vi "Setting.vi"() -> ()   [LabVIEW 2020]
uses:
  Libraries/S7/S7.lvlib
  <userlib>/_MGI/1D Array/MGI Average/MGI Average (DBL[]).vi
panel:
  in  "输出轴大量程标定":bool
  in  "停止":bool
  in  "输出轴小量程标定":bool
  in  "输入轴标定":bool
  out "标定曲线":cluster{dbl[], dbl[]}[](graph)
  # "配置标定"
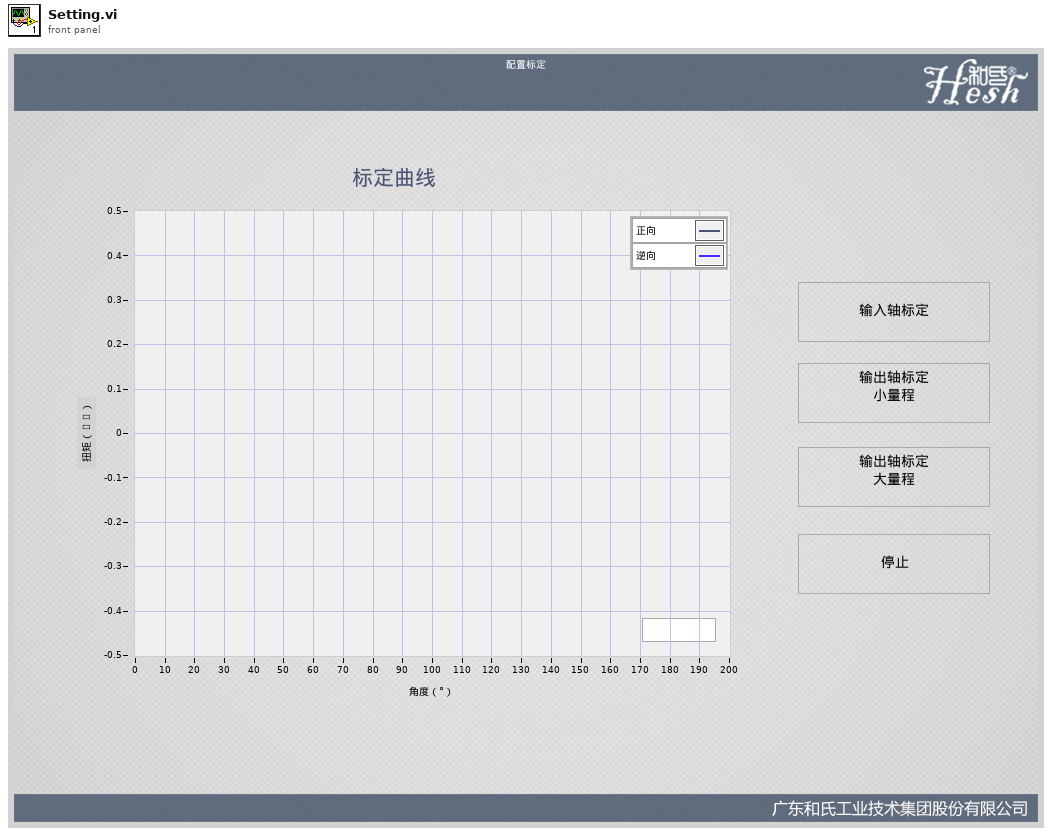
[diagram p1: front panel]
types:
  T1 = cluster{"输入旋转位移":sgl, "输入移载位移":sgl, "工装移载位移":sgl, "输入编码位移":sgl, "输入扭矩":sgl, "输出扭矩(小)":sgl, "输出扭矩(大)":sgl, "吸收电流":sgl}
  T2 = cluster{"输入轴扭矩":dbl, "输出轴扭矩小量程":dbl, "输出轴扭矩大量程":dbl}
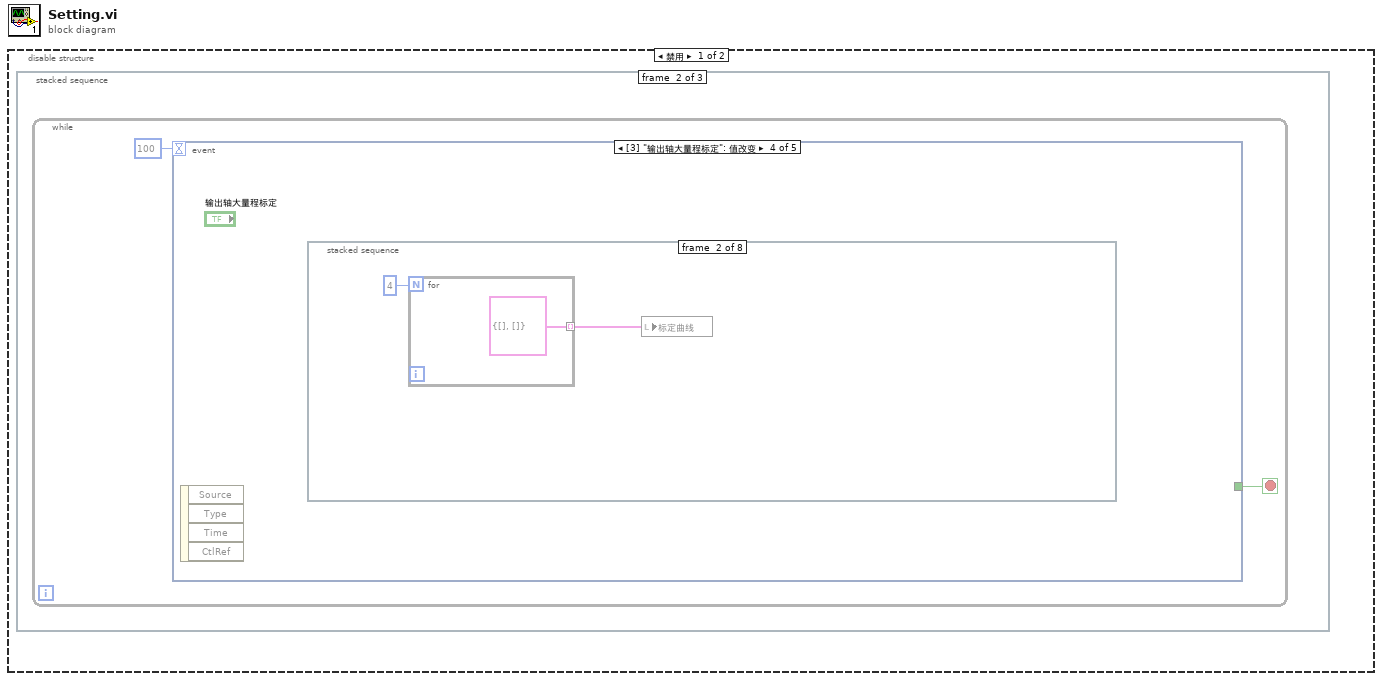
[diagram p0: block diagram]
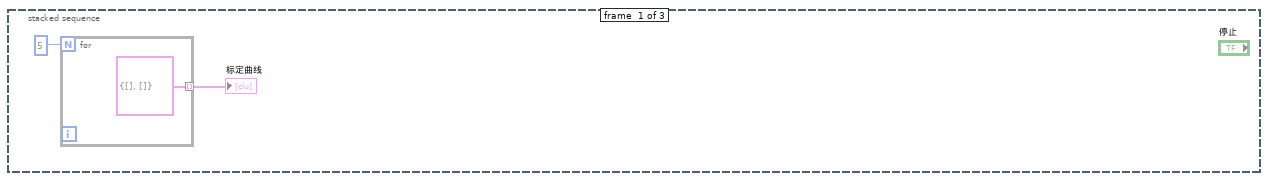
[diagram p2: hidden frame]
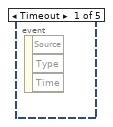
[diagram p3: hidden frame]
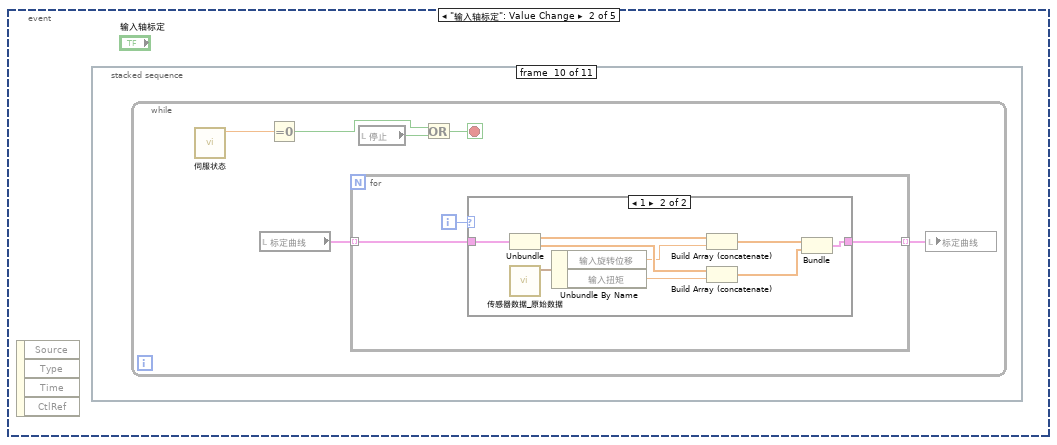
[diagram p4: hidden frame]
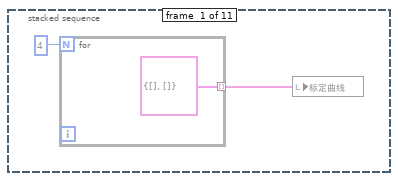
[diagram p5: hidden frame]
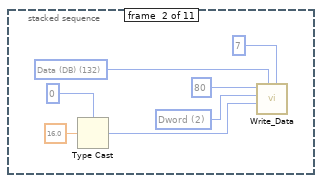
[diagram p6: hidden frame]
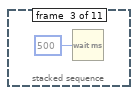
[diagram p7: hidden frame]
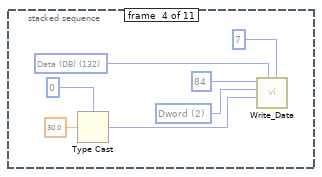
[diagram p8: hidden frame]
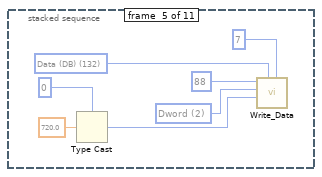
[diagram p9: hidden frame]
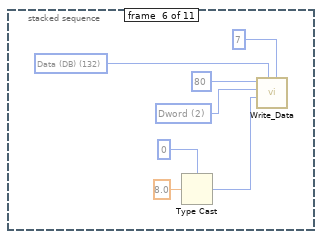
[diagram p10: hidden frame]
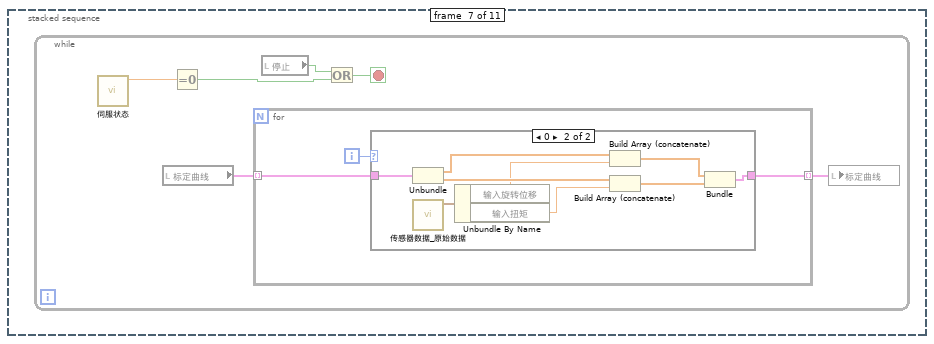
[diagram p11: hidden frame]
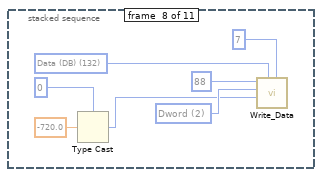
[diagram p13: hidden frame]
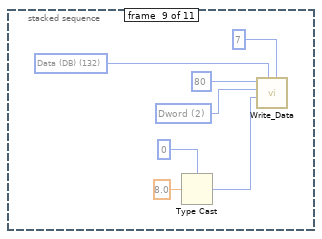
[diagram p14: hidden frame]
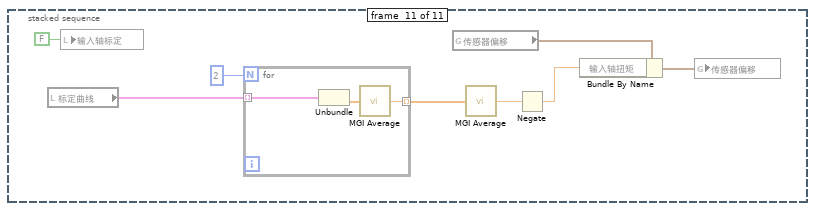
[diagram p16: hidden frame]
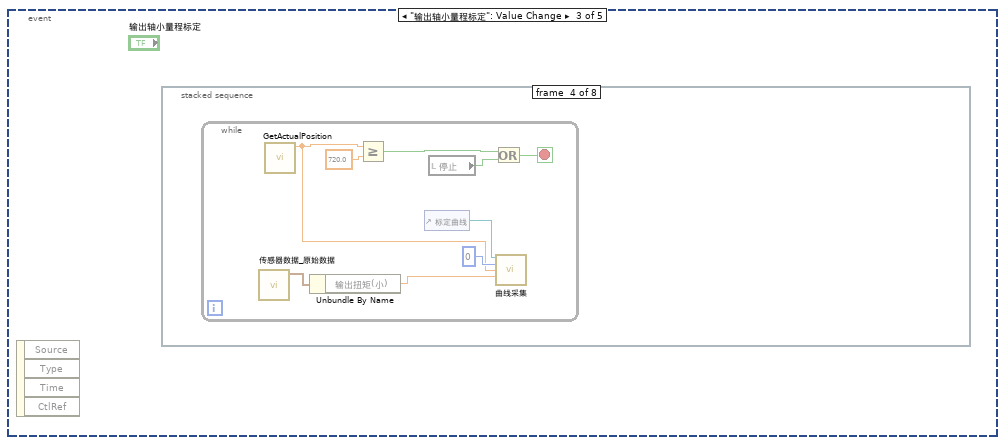
[diagram p17: hidden frame]
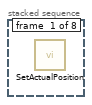
[diagram p18: hidden frame]
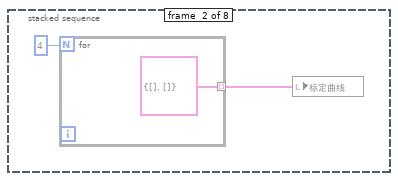
[diagram p19: hidden frame]
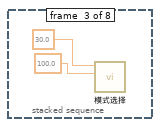
[diagram p20: hidden frame]
diagram:
  n1 = disable-structure shown="禁用" {
    frame Disabled {
      n2 = stacked-sequence {
        frame #0 {
          n3 = for {
            N: 5 -> [_]
            tunnel: [cluster{dbl[], dbl[]} {[], []}] -> w1 mode=indexing
          }
          "标定曲线" <- w1
        }
        frame #1 {
          n4 = while {
            stop <- w5 stop-if-true
            n5 = event shown="[3] \"输出轴大量程标定\": 值改变" {
              selector: _ -> [_ _ _ _ _]
              dyn-events: _ -> [_ _ _ _ _]
              timeout: 100 -> [_ _ _ _ _]
              tunnel: [_ _ _ _ TRUE] -> w5
              event Timeout {
                n6 = event-data() -> ()  [unwired: 1 in, 3 out]
              }
              event "输入轴标定": Value Change {
                n7 = event-data() -> ()  [unwired: 1 in, 4 out]
                n8 = stacked-sequence {
                  frame #0 {
                    n9 = for {
                      N: 4 -> [_]
                      tunnel: [cluster{dbl[], dbl[]} {[], []}] -> w7 mode=indexing
                    }
                    n10 = local write "标定曲线"(w7) -> ()
                  }
                  frame #1 {
                    w13 = u16 2 items=["byte", "word", "Dword"] ("数据类型")
                    w15 = u8 132 items=["I/O (P)"=128, "Input (I)"=129, "Output (Q)"=130, "Bit Memory (M)"=131, "Data (DB)"=132, "Instance Data (DI)"=133, "Local Data (L)"=134, "Predecessor Local Data (VL)"=135] ("寄存器类型")
                    n11 = Type Cast(type=u32 0, x=sgl 16.0 ("输入轴旋转绝对位置")) -> (*(type *) &x=w11:u32)
                    n12 = call "Write_Data.vi"("DB #"=u16 7, "寄存器类型"=w15, "写入数据"=w11, "数据类型"=w13, "写入地址"=u32 80) -> ()  [unwired: 4 in, 3 out]
                  }
                  frame #2 {
                    n13 = Wait (ms)(milliseconds to wait=u32 500 ("等待时间（毫秒）")) -> ()  [unwired: 1 out]
                  }
                  frame #3 {
                    w21 = u16 2 items=["byte", "word", "Dword"] ("数据类型")
                    w23 = u8 132 items=["I/O (P)"=128, "Input (I)"=129, "Output (Q)"=130, "Bit Memory (M)"=131, "Data (DB)"=132, "Instance Data (DI)"=133, "Local Data (L)"=134, "Predecessor Local Data (VL)"=135] ("寄存器类型")
                    n14 = Type Cast(type=u32 0, x=sgl 30.0 ("输入轴旋转绝对位置")) -> (*(type *) &x=w19:u32)
                    n15 = call "Write_Data.vi"("DB #"=u16 7, "寄存器类型"=w23, "写入数据"=w19, "数据类型"=w21, "写入地址"=u32 84) -> ()  [unwired: 4 in, 3 out]
                  }
                  frame #4 {
                    w27 = u16 2 items=["byte", "word", "Dword"] ("数据类型")
                    w28 = u8 132 items=["I/O (P)"=128, "Input (I)"=129, "Output (Q)"=130, "Bit Memory (M)"=131, "Data (DB)"=132, "Instance Data (DI)"=133, "Local Data (L)"=134, "Predecessor Local Data (VL)"=135] ("寄存器类型")
                    n16 = Type Cast(type=u32 0, x=sgl 720.0 ("输入轴旋转绝对位置")) -> (*(type *) &x=w30:u32)
                    n17 = call "Write_Data.vi"("DB #"=u16 7, "寄存器类型"=w28, "写入数据"=w30, "数据类型"=w27, "写入地址"=u32 88) -> ()  [unwired: 4 in, 3 out]
                  }
                  frame #5 {
                    w34 = u16 2 items=["byte", "word", "Dword"] ("数据类型")
                    w35 = u8 132 items=["I/O (P)"=128, "Input (I)"=129, "Output (Q)"=130, "Bit Memory (M)"=131, "Data (DB)"=132, "Instance Data (DI)"=133, "Local Data (L)"=134, "Predecessor Local Data (VL)"=135] ("寄存器类型")
                    n18 = Type Cast(type=u32 0, x=sgl 8.0 ("输入轴旋转绝对位置")) -> (*(type *) &x=w37:u32)
                    n19 = call "Write_Data.vi"("DB #"=u16 7, "寄存器类型"=w35, "写入数据"=w37, "数据类型"=w34, "写入地址"=u32 80) -> ()  [unwired: 4 in, 3 out]
                  }
                  frame #6 {
                    n20 = while {
                      stop <- w42 stop-if-true
                      n21 = call "伺服状态.vi"() -> ("Status"=w39:sgl)  [unwired: 11 in]
                      n22 = local read "标定曲线"() -> (w41:cluster{dbl[], dbl[]}[])
                      n23 = Equal To 0?(x=w39) -> (x = 0?=w38:bool)
                      n24 = for {
                        tunnel: [w44] -> w40 mode=indexing
                        tunnel: w41 -> [w46] mode=indexing
                        i -> [w45]
                        n25 = case shown="0" w45 {
                          tunnel: [w47 w51] -> w44
                          tunnel: w46 -> [w47 w52]
                          frame Default {
                          }
                          frame 0 {
                            n26 = Unbundle(w52) -> (w56:dbl[], w55:dbl[])
                            n27 = call "传感器数据_原始数据.vi"() -> ("传感器读数"=w50:T1)  [unwired: 11 in]
                            n28 = Unbundle By Name(w50) -> ("输入旋转位移"=w49:sgl, "输入扭矩"=w48:sgl)
                            n29 = Build Array (concatenate)(w56, w49) -> (w54:dbl[])
                            n30 = Build Array (concatenate)(w55, w48) -> (w53:dbl[])
                            n31 = Bundle(w54, w53) -> (w51:cluster{dbl[], dbl[]})  [unwired: 1 in]
                          }
                        }
                      }
                      n32 = local read "停止"() -> (w43:bool)
                      n33 = Or(x=w43, y=w38) -> (x .or. y?=w42:bool)
                      n34 = local write "标定曲线"(w40) -> ()
                    }
                  }
                  frame #7 {
                    w61 = u16 2 items=["byte", "word", "Dword"] ("数据类型")
                    w63 = u8 132 items=["I/O (P)"=128, "Input (I)"=129, "Output (Q)"=130, "Bit Memory (M)"=131, "Data (DB)"=132, "Instance Data (DI)"=133, "Local Data (L)"=134, "Predecessor Local Data (VL)"=135] ("寄存器类型")
                    n35 = Type Cast(type=u32 0, x=sgl -720.0 ("输入轴旋转绝对位置")) -> (*(type *) &x=w59:u32)
                    n36 = call "Write_Data.vi"("DB #"=u16 7, "寄存器类型"=w63, "写入数据"=w59, "数据类型"=w61, "写入地址"=u32 88) -> ()  [unwired: 4 in, 3 out]
                  }
                  frame #8 {
                    w68 = u16 2 items=["byte", "word", "Dword"] ("数据类型")
                    w70 = u8 132 items=["I/O (P)"=128, "Input (I)"=129, "Output (Q)"=130, "Bit Memory (M)"=131, "Data (DB)"=132, "Instance Data (DI)"=133, "Local Data (L)"=134, "Predecessor Local Data (VL)"=135] ("寄存器类型")
                    n37 = Type Cast(type=u32 0, x=sgl 8.0 ("输入轴旋转绝对位置")) -> (*(type *) &x=w66:u32)
                    n38 = call "Write_Data.vi"("DB #"=u16 7, "寄存器类型"=w70, "写入数据"=w66, "数据类型"=w68, "写入地址"=u32 80) -> ()  [unwired: 4 in, 3 out]
                  }
                  frame #9 {
                    n39 = while {
                      stop <- w76 stop-if-true
                      n40 = call "伺服状态.vi"() -> ("Status"=w72:sgl)  [unwired: 11 in]
                      n41 = local read "标定曲线"() -> (w74:cluster{dbl[], dbl[]}[])
                      n42 = Equal To 0?(x=w72) -> (x = 0?=w71:bool)
                      n43 = for {
                        tunnel: [w77] -> w73 mode=indexing
                        tunnel: w74 -> [w79] mode=indexing
                        i -> [w78]
                        n44 = case shown="1" w78 {
                          tunnel: [w80 w84] -> w77
                          tunnel: w79 -> [w80 w85]
                          frame Default {
                          }
                          frame 1 {
                            n45 = Unbundle(w85) -> (w89:dbl[], w88:dbl[])
                            n46 = call "传感器数据_原始数据.vi"() -> ("传感器读数"=w83:T1)  [unwired: 11 in]
                            n47 = Unbundle By Name(w83) -> ("输入旋转位移"=w81:sgl, "输入扭矩"=w82:sgl)
                            n48 = Build Array (concatenate)(w89, w81) -> (w87:dbl[])
                            n49 = Build Array (concatenate)(w88, w82) -> (w86:dbl[])
                            n50 = Bundle(w87, w86) -> (w84:cluster{dbl[], dbl[]})  [unwired: 1 in]
                          }
                        }
                      }
                      n51 = local read "停止"() -> (w75:bool)
                      n52 = Or(x=w71, y=w75) -> (x .or. y?=w76:bool)
                      n53 = local write "标定曲线"(w73) -> ()
                    }
                  }
                  frame #10 {
                    n54 = local read "标定曲线"() -> (w90:cluster{dbl[], dbl[]}[])
                    n55 = local write "输入轴标定"(FALSE ("输入轴标定")) -> ()
                    n56 = for {
                      N: 2 -> [_]
                      tunnel: w90 -> [w100] mode=indexing
                      tunnel: [w98] -> w92 mode=indexing
                      n57 = Unbundle(w100) -> (w99:dbl[])  [unwired: 1 out]
                      n58 = call-poly <userlib>:"MGI Average.vi"("Double[]"=w99) -> ("Average"=w98:dbl)  [unwired: 1 in]
                    }
                    n59 = global read "传感器偏移.vi" "传感器偏移"() -> (w94:T2)
                    n60 = call-poly <userlib>:"MGI Average.vi"("Double[]"=w92) -> ("Average"=w96:dbl)  [unwired: 1 in]
                    n61 = Negate(x=w96) -> (-x=w91:dbl)
                    n62 = Bundle By Name(cluster=w94, "输入轴扭矩"=w91) -> (w95:T2)
                    n63 = global write "传感器偏移.vi" "传感器偏移"(w95) -> ()
                  }
                }
              }
              event "输出轴小量程标定": Value Change {
                n64 = event-data() -> ()  [unwired: 1 in, 4 out]
                n65 = stacked-sequence {
                  frame #0 {
                    n66 = call "SetActualPosition.vi"() -> ()  [unwired: 11 in, 1 out]
                  }
                  frame #1 {
                    n67 = for {
                      N: 4 -> [_]
                      tunnel: [cluster{dbl[], dbl[]} {[], []}] -> w102 mode=indexing
                    }
                    n68 = local write "标定曲线"(w102) -> ()
                  }
                  frame #2 {
                    n69 = call-poly "模式选择.vi"("Max Torque"=100.0, "Velocity"=30.0) -> ()  [unwired: 9 in, 1 out]
                  }
                  frame #3 {
                    n70 = while {
                      stop <- w106 stop-if-true
                      n71 = call "传感器数据_原始数据.vi"() -> ("传感器读数"=w114:T1)  [unwired: 11 in]
                      n72 = call "GetActualPosition.vi"() -> ("Axis_ActualPosition(°)"=w109:dbl)  [unwired: 11 in]
                      n73 = Unbundle By Name(w114) -> ("输出扭矩(小)"=w111:sgl)
                      n74 = Greater Or Equal?(x=w109, y=720.0) -> (x >= y?=w107:bool)
                      n75 = control-ref of="标定曲线"() -> (w112:refnum<vi>)
                      n76 = local read "停止"() -> (w110:bool)
                      n77 = Or(x=w107, y=w110) -> (x .or. y?=w106:bool)
                      n78 = call "曲线采集.vi"("曲线引用"=w112, "曲线索引"=0, "X"=w109, "Y"=w111) -> ()  [unwired: 10 in, 2 out]
                    }
                  }
                  frame #4 {
                    n79 = call-poly "模式选择.vi"("Max Torque"=100.0, "Velocity"=-30.0) -> ()  [unwired: 9 in, 1 out]
                  }
                  frame #5 {
                    n80 = while {
                      stop <- w117 stop-if-true
                      n81 = call "传感器数据_原始数据.vi"() -> ("传感器读数"=w125:T1)  [unwired: 11 in]
                      n82 = call "GetActualPosition.vi"() -> ("Axis_ActualPosition(°)"=w120:dbl)  [unwired: 11 in]
                      n83 = Unbundle By Name(w125) -> ("输出扭矩(小)"=w122:sgl)
                      n84 = Less Or Equal?(x=w120, y=0.0) -> (x <= y?=w118:bool)
                      n85 = control-ref of="标定曲线"() -> (w123:refnum<vi>)
                      n86 = local read "停止"() -> (w121:bool)
                      n87 = Or(x=w118, y=w121) -> (x .or. y?=w117:bool)
                      n88 = call "曲线采集.vi"("曲线引用"=w123, "曲线索引"=1, "X"=w120, "Y"=w122) -> ()  [unwired: 10 in, 2 out]
                    }
                  }
                  frame #6 {
                    n89 = local write "输出轴小量程标定"(FALSE ("输入轴标定")) -> ()
                    n90 = call-poly "模式选择.vi"() -> ()  [unwired: 11 in, 1 out]
                  }
                  frame #7 {
                    n91 = local read "标定曲线"() -> (w127:cluster{dbl[], dbl[]}[])
                    n92 = for {
                      N: 2 -> [_]
                      tunnel: w127 -> [w135] mode=indexing
                      tunnel: [w133] -> w128 mode=indexing
                      n93 = Unbundle(w135) -> (w134:dbl[])  [unwired: 1 out]
                      n94 = call-poly <userlib>:"MGI Average.vi"("Double[]"=w134) -> ("Average"=w133:dbl)  [unwired: 1 in]
                    }
                    n95 = global read "传感器偏移.vi" "传感器偏移"() -> (w130:T2)
                    n96 = call-poly <userlib>:"MGI Average.vi"("Double[]"=w128) -> ("Average"=w132:dbl)  [unwired: 1 in]
                    n97 = Bundle By Name(cluster=w130, "输出轴扭矩小量程"=w132) -> (w131:T2)
                    n98 = global write "传感器偏移.vi" "传感器偏移"(w131) -> ()
                  }
                }
              }
              event "输出轴大量程标定": Value Change {
                n99 = event-data() -> ()  [unwired: 1 in, 4 out]
                n100 = stacked-sequence {
                  frame #0 {
                    n101 = call "SetActualPosition.vi"() -> ()  [unwired: 11 in, 1 out]
                  }
                  frame #1 {
                    n102 = for {
                      N: 4 -> [_]
                      tunnel: [cluster{dbl[], dbl[]} {[], []}] -> w137 mode=indexing
                    }
                    n103 = local write "标定曲线"(w137) -> ()
                  }
                  frame #2 {
                    n104 = call-poly "模式选择.vi"("Max Torque"=100.0, "Velocity"=30.0) -> ()  [unwired: 9 in, 1 out]
                  }
                  frame #3 {
                    n105 = while {
                      stop <- w141 stop-if-true
                      n106 = call "GetActualPosition.vi"() -> ("Axis_ActualPosition(°)"=w144:dbl)  [unwired: 11 in]
                      n107 = call "传感器数据_原始数据.vi"() -> ("传感器读数"=w149:T1)  [unwired: 11 in]
                      n108 = Unbundle By Name(w149) -> ("输出扭矩(大)"=w146:sgl)
                      n109 = Greater Or Equal?(x=w144, y=720.0) -> (x >= y?=w142:bool)
                      n110 = control-ref of="标定曲线"() -> (w148:refnum<vi>)
                      n111 = local read "停止"() -> (w145:bool)
                      n112 = Or(x=w142, y=w145) -> (x .or. y?=w141:bool)
                      n113 = call "曲线采集.vi"("曲线引用"=w148, "曲线索引"=0, "X"=w144, "Y"=w146) -> ()  [unwired: 10 in, 2 out]
                    }
                  }
                  frame #4 {
                    n114 = call-poly "模式选择.vi"("Max Torque"=100.0, "Velocity"=-30.0) -> ()  [unwired: 9 in, 1 out]
                  }
                  frame #5 {
                    n115 = while {
                      stop <- w153 stop-if-true
                      n116 = call "传感器数据_原始数据.vi"() -> ("传感器读数"=w160:T1)  [unwired: 11 in]
                      n117 = call "GetActualPosition.vi"() -> ("Axis_ActualPosition(°)"=w156:dbl)  [unwired: 11 in]
                      n118 = Unbundle By Name(w160) -> ("输出扭矩(大)"=w152:sgl)
                      n119 = Less Or Equal?(x=w156, y=0.0) -> (x <= y?=w154:bool)
                      n120 = control-ref of="标定曲线"() -> (w158:refnum<vi>)
                      n121 = local read "停止"() -> (w157:bool)
                      n122 = Or(x=w154, y=w157) -> (x .or. y?=w153:bool)
                      n123 = call "曲线采集.vi"("曲线引用"=w158, "曲线索引"=1, "X"=w156, "Y"=w152) -> ()  [unwired: 10 in, 2 out]
                    }
                  }
                  frame #6 {
                    n124 = local write "输出轴大量程标定"(FALSE ("输入轴标定")) -> ()
                    n125 = call-poly "模式选择.vi"() -> ()  [unwired: 11 in, 1 out]
                  }
                  frame #7 {
                    n126 = local read "标定曲线"() -> (w162:cluster{dbl[], dbl[]}[])
                    n127 = for {
                      N: 2 -> [_]
                      tunnel: w162 -> [w170] mode=indexing
                      tunnel: [w168] -> w163 mode=indexing
                      n128 = Unbundle(w170) -> (w169:dbl[])  [unwired: 1 out]
                      n129 = call-poly <userlib>:"MGI Average.vi"("Double[]"=w169) -> ("Average"=w168:dbl)  [unwired: 1 in]
                    }
                    n130 = global read "传感器偏移.vi" "传感器偏移"() -> (w165:T2)
                    n131 = call-poly <userlib>:"MGI Average.vi"("Double[]"=w163) -> ("Average"=w167:dbl)  [unwired: 1 in]
                    n132 = Bundle By Name(cluster=w165, "输出轴扭矩大量程"=w167) -> (w166:T2)
                    n133 = global write "传感器偏移.vi" "传感器偏移"(w166) -> ()
                  }
                }
              }
              event Panel Close {
                n134 = event-data() -> ()  [unwired: 1 in, 4 out]
              }
            }
          }
        }
        frame #2 {
          n135 = global read "传感器偏移.vi" "传感器偏移"() -> (w173:T2)
          n136 = call "Demarcate.vi"("Mode"=enum16{"Read", "Write"}."Write", "Sensor IN"=w173) -> ()  [unwired: 8 in, 2 out]
        }
      }
    }
    frame Enabled {
    }
  }
